vi "W2Q2.vi"(1 "Numeric 2":dbl) -> (0 "Numeric":i32)   [LabVIEW 2023]
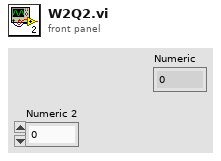
[diagram p1: front panel]
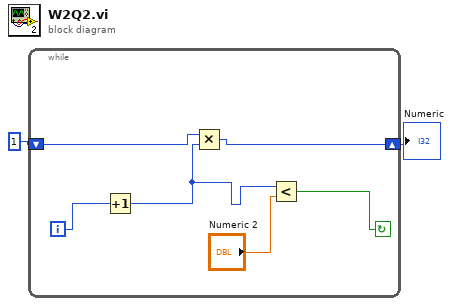
[diagram p0: block diagram]
diagram:
  n1 = while {
    shift-right: [w7] -> w1
    shift-left: 1 -> [w8]
    i -> [w6]
    stop <- w4 continue-if-true
    n2 = Increment(x=w6) -> (x+1=w5:i32)
    n3 = Multiply(x=w8, y=w5) -> (x*y=w7:i32)
    n4 = Less?(x=w5, y="Numeric 2") -> (x < y?=w4:bool)
  }
  "Numeric" <- w1
